vi "Switch Counter Signal For Auto.vi"(8 "error in (no error)":errorcluster, 9 "Protected Signal GUID":string="D95BE1B9-793B-430A-998F-7F352C03EC7C", 10 "Counter Value GUID":string="94e87467-031b-484c-a85e-bcbac581524d", 11 "Node Ptr":T1 format="%.0x") -> (0 "error out":errorcluster)   [LabVIEW 2023, in "Protection and Counter Support System Explorer.lvlib"]
uses:
  Protection and Counter Support System Explorer.lvlib
  <vilib>/NI VeriStand/Custom Device API/Custom Device Item Ref.ctl
  <vilib>/NI VeriStand/Custom Device API/Custom Device API.lvlib
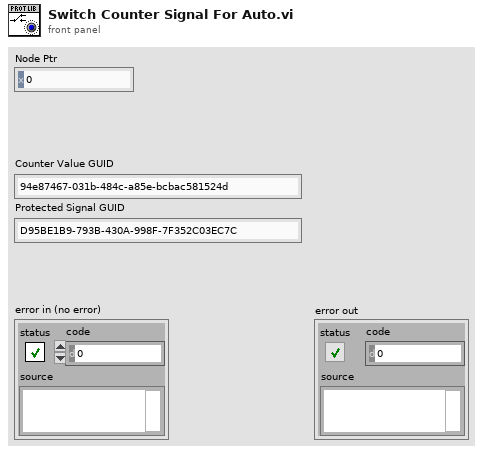
[diagram p1: front panel]
types:
  T1 = typedef "Custom Device API.lvlib/Custom Device Item Ref.ctl" = u64
  T2 = typedef "Custom Device API.lvlib/Custom Device Item Info.ctl" = cluster{"Name":string, "Is Channel":bool, "GUID":string, "Is Waveform":bool}
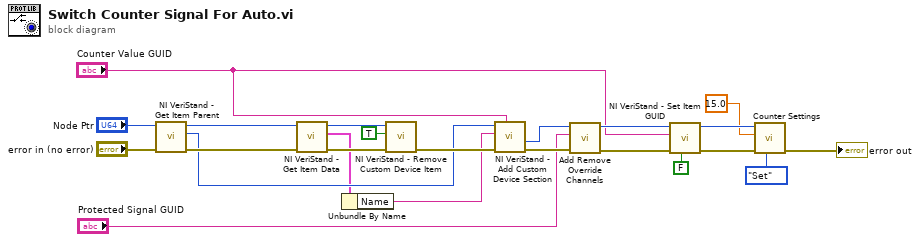
[diagram p0: block diagram]
diagram:
  n1 = call <vilib>:"NI VeriStand - Get Item Parent.vi"("error in (no error)"="error in (no error)", "Item Ref in"="Node Ptr") -> ("error out"=w18:errorcluster, "Parent Ref"=w16:T1, "Item Ref out"=w19:T1)  [unwired: 6 in, 1 out]
  n2 = call <vilib>:"NI VeriStand - Get Item Data.vi"("error in (no error)"=w18, "Item Ref in"=w19) -> ("error out"=w14:errorcluster, "Item Info"=w13:T2, "Item Ref out"=w15:T1)  [unwired: 6 in, 1 out]
  n3 = Unbundle By Name(w13) -> ("Name"=w12:string)
  n4 = call <vilib>:"NI VeriStand - Remove Custom Device Item.vi"("error in (no error)"=w14, "Force Delete (F)"=TRUE, "Item Ref in"=w15) -> ("error out"=w17:errorcluster)  [unwired: 7 in, 1 out]
  n5 = call <vilib>:"NI VeriStand - Add Custom Device Section.vi"("GUID (Default Section)"="Counter Value GUID", "error in (no error)"=w17, "Section Name"=w12, "Parent Ref in"=w16) -> ("error out"=w8:errorcluster, "Section Ptr"=w9:T1)  [unwired: 4 in, 2 out]
  n6 = call "Add Remove Override Channels.vi"("error in (no error)"=w8, "Protected Signal GUID"="Protected Signal GUID", "Channel Ref in"=w9) -> ("error out"=w22:errorcluster, "Channel Ref out"=w23:T1)  [unwired: 7 in]
  n7 = call <vilib>:"NI VeriStand - Set Item GUID.vi"("Refresh System Explorer Tree? (F)"=FALSE, "error in (no error)"=w22, "GUID"="Counter Value GUID", "Item Ref in"=w23) -> ("error out"=w6:errorcluster, "Item Ref out"=w4:T1)  [unwired: 6 in]
  n8 = call "Counter Settings.vi"("Action"=enum8{"Get", "Set"}."Set", "error in"=w6, "Max Count"=15.0, "Parent Ref"=w4) -> ("error out"=→"error out":errorcluster)  [unwired: 5 in, 2 out]
